vi "Setup Check Labels Only (SubVI).vi"(3 "error in (no error)":errorcluster, 4 "[error source] (\" \")":string, 5 "Labels Array":string[](array[string])) -> (9 "Cluster Array Out":cluster{"Label":string}[](array[cluster]), 10 "error out":errorcluster)   [LabVIEW 2011]
uses:
  <vilib>/Utility/error.llb/DialogType.ctl
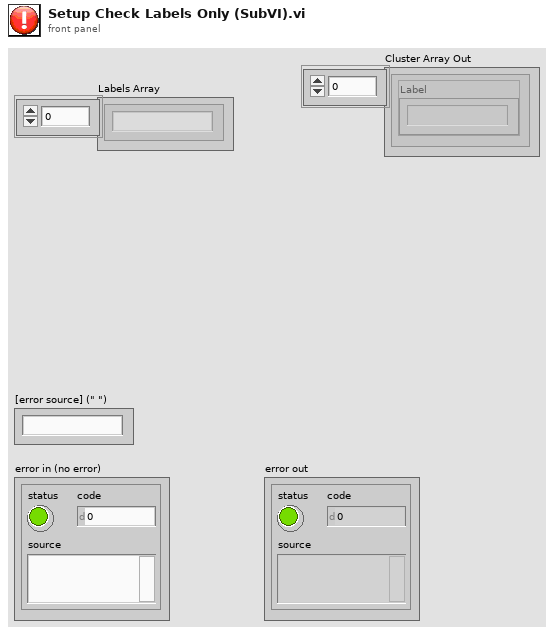
[diagram p1: front panel]
types:
  T1 = typedef "DialogType.ctl" = u16
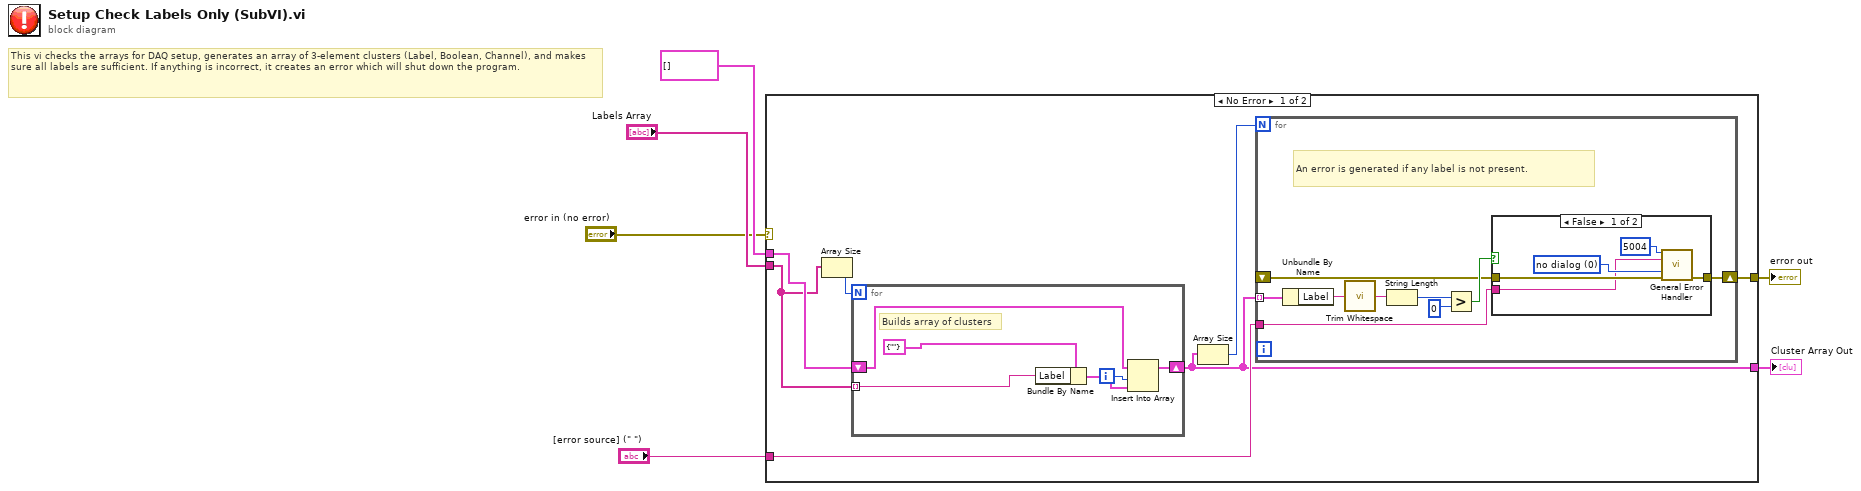
[diagram p0: block diagram]
diagram:
  # "This vi checks the arrays for DAQ setup, generates an array of 3-element clusters (Label, Boolean, Channel), and makes sure all labels are sufficient. If anything is incorrect, it creates an error which will shut down the program."
  n1 = case shown="No Error" "error in (no error)" {
    selector: "error in (no error)" -> [_ w35]
    tunnel: "Labels Array" -> [w7 _]
    tunnel: [w10 w35] -> w4
    tunnel: "[error source] (\" \")" -> [w11 _]
    tunnel: cluster{"Label":string}[] [] -> [w8 w36]
    tunnel: [w9 w36] -> w1
    frame No Error {
      n2 = Array Size(array=w7) -> (size(s)=w13:i32)
      n3 = for {
        N: w13 -> [_]
        tunnel: w7 -> [w34] mode=indexing
        shift-right: [w32] -> w9
        shift-left: w8 -> [w31]
        i -> [w30]
        # "Builds array of clusters"
        n4 = Bundle By Name(cluster=cluster{"Label":string} {"Label"=""}, "Label"=w34) -> (w33:cluster{"Label":string})
        n5 = Insert Into Array(array=w31, index=w30, new element=w33) -> (w32:cluster{"Label":string}[])
      }
      n6 = Array Size(array=w9) -> (size(s)=w12:i32)
      n7 = for {
        N: w12 -> [_]
        tunnel: w9 -> [w22] mode=indexing
        shift-right: [w15] -> w10
        shift-left: _ -> [w16]
        tunnel: w11 -> [w14]
        # "An error is generated if any label is not present."
        n8 = Unbundle By Name(w22) -> ("Label"=w21:string)
        n9 = call <vilib>:"Trim Whitespace.vi"("string"=w21) -> ("trimmed string"=w20:string)  [unwired: 1 in]
        n10 = String Length(string=w20) -> (length=w19:i32)
        n11 = Greater?(x=w19, y=0) -> (0:w17:bool)
        n12 = case shown="False" w17 {
          tunnel: w16 -> [w25 w28]
          tunnel: [w24 w28] -> w15
          tunnel: w14 -> [w23 _]
          frame False {
            w26 = T1 0 items=["no dialog", "OK message", "continue or stop message", "OK message + warnings", "continue/stop + warnings"] ("type of dialog (OK msg:1)")
            n13 = call <vilib>:"General Error Handler.vi"("[error code] (0)"=5004, "[error source] (\" \")"=w23, "type of dialog (OK msg:1)"=w26, "error in (no error)"=w25) -> ("error out"=w24:errorcluster)  [unwired: 7 in, 4 out]
          }
          frame True {
          }
        }
      }
    }
    frame Error {
    }
  }
  "error out" <- w4
  "Cluster Array Out" <- w1
